vi "Joystick_Buttons.vi"() -> ()   [LabVIEW 2019]
panel:
  out "right-LeftArrayBL":bool
  out "right-LeftArrayBM":bool
  out "right-LeftArrayBR":bool
  out "right-LeftArrayTR":bool
  out "right-LeftArrayTM":bool
  out "right-LeftArrayTL":bool
  out "left-LeftArrayBL":bool
  out "left-LeftArrayBM":bool
  out "left-LeftArrayBR":bool
  out "left-LeftArrayTR":bool
  out "left-LeftArrayTM":bool
  out "left-LeftArrayTL":bool
  in  "rightSlider":dbl
  in  "rightZ":dbl
  in  "rightY":dbl
  in  "rightX":dbl
  in  "leftSlider":dbl
  in  "leftZ":dbl
  in  "leftY":dbl
  in  "leftX":dbl
  out "right-RightArrayBR":bool
  out "right-RightArrayBM":bool
  out "right-RightArrayBL":bool
  out "right-RightArrayTL":bool
  out "right-RightArrayTM":bool
  out "right-RightArrayTR":bool
  out "right-ThumbR":bool
  out "right-ThumbL":bool
  out "right-ThumbMain":bool
  out "right-Trigger":bool
  out "left-RightArrayBR":bool
  out "left-RightArrayBM":bool
  out "left-RightArrayBL":bool
  out "left-RightArrayTL":bool
  out "left-RightArrayTM":bool
  out "left-RightArrayTR":bool
  out "left-ThumbR":bool
  out "left-ThumbL":bool
  out "left-ThumbMain":bool
  out "left-Trigger":bool
  # "Left Joystick"
  # "Right Joystick"
  # "Axes Left"
  # "Axes Left"
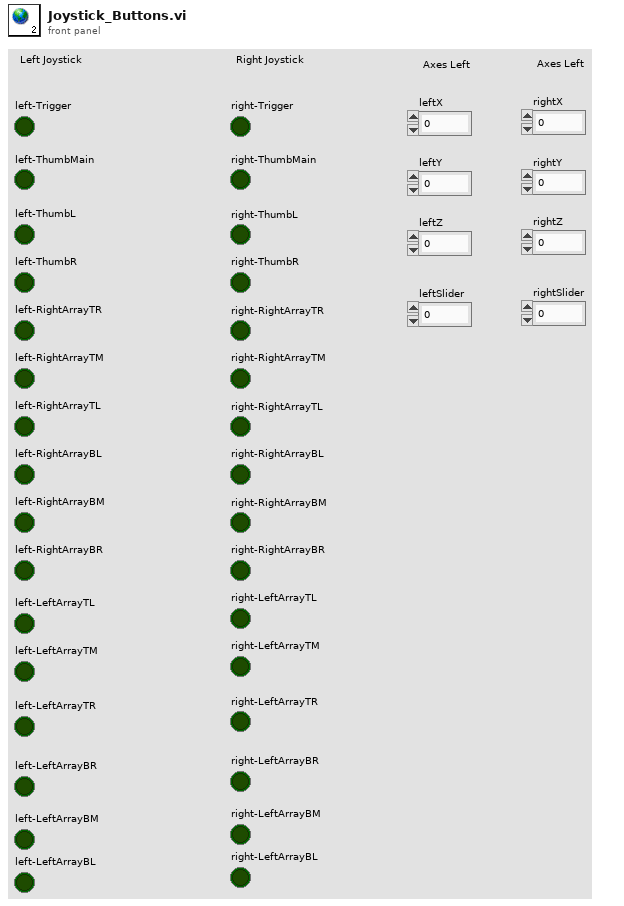
[diagram p1: front panel]
diagram:
